vi "Set Output State.vi"(8 "error in (no error)":cluster{"状态":bool, "代码":i32, "源":string} caption="错误输入（无错误）", 10 "输出状态":bool, 11 "仿真水位":refnum<class "Simulated Water Level.lvclass">) -> (0 "error out":cluster{"状态":bool, "代码":i32, "源":string} caption="错误输出", 3 "仿真水位":refnum<class "Simulated Water Level.lvclass">)   [LabVIEW 2015, in "Simulated Water Level.lvclass"]
doc: "该VI负责在水位控制器所监控的变量值高于或低于死区范围时，设定水位控制器的行为。仅当操作模式发生切换时，该VI由水位控制器类调用。\n\n在水位控制器类中，该VI指定水位低于死区阈值时，打开阀门。液罐中重新注水之后，阀门再次关闭。"
uses:
  Simulated Water Level.lvclass
  Cooler Plug-Ins/Simulated Evaporative Cooler.lvclass/Simulation Data_Global.vi
  Cooler Plug-Ins/Simulated Evaporative Cooler.lvclass/Simulated Evaporative Cooler.lvclass
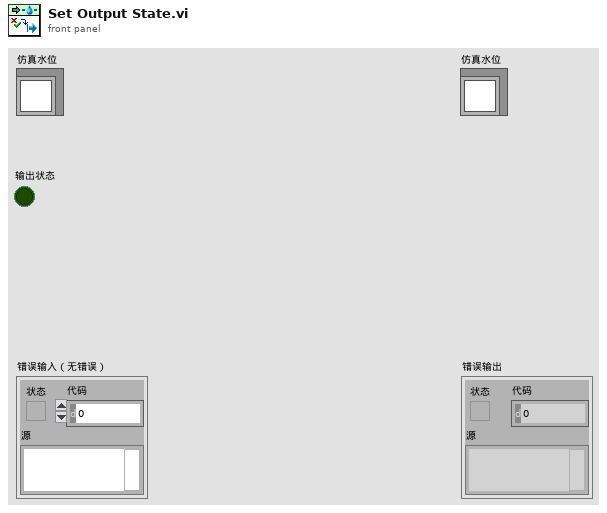
[diagram p1: front panel]
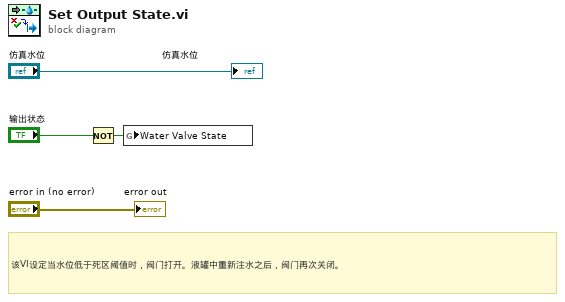
[diagram p0: block diagram]
diagram:
  # "该VI设定当水位低于死区阈值时，阀门打开。液罐中重新注水之后，阀门再次关闭。"
  n1 = Not(x="输出状态") -> (.not. x?=w2:bool)
  n2 = global write "Simulation Data_Global.vi" "Water Valve State"(w2) -> ()
  "error out" <- "error in (no error)"
  "仿真水位" <- "仿真水位"
